vi "3-Position Solenoid Control.vi"(6 "Sensor Analog Status":sgl format="%#_13g", 7 "Sensor Digital Status":bool, 9 "Feedback":T5, 10 "Action":T4(ring), 11 "PneumaticsDevRefIn":T1={"Pneumatic State Reference"=refnum, "SolenoidDevRef"={"DevStatus"={"status"=FALSE, "code"=0, "source"=""}, "Pneumatics Control Module"=0, "Forward Solenoid Channel"=enum."Invalid", "Reverse Solenoid Channel"=enum."Invalid"}, "Pneumatic Configuration reference"=refnum}) -> (1 "Action Complete":bool, 2 "Forward":bool, 3 "PneumaticsDevRefOut":T1={"Pneumatic State Reference"=refnum, "SolenoidDevRef"={"DevStatus"={"status"=FALSE, "code"=0, "source"=""}, "Pneumatics Control Module"=0, "Forward Solenoid Channel"=enum."Invalid", "Reverse Solenoid Channel"=enum."Invalid"}, "Pneumatic Configuration reference"=refnum})   [LabVIEW 2015]
uses:
  <userlib>/836 Library/Pneumatics/Common/Feedback Typedef.ctl
  <userlib>/836 Library/Pneumatics/Pneumatics/836_PneumaticsDevRef.ctl
  <userlib>/836 Library/Pneumatics/Pneumatics/Pneumatic State.ctl
  <userlib>/836 Library/Pneumatics/Pneumatics/StateMachine.ctl
  <vilib>/Rock Robotics/WPI/Solenoid/WPI_SolenoidDevRef.ctl
  <vilib>/Rock Robotics/WPI/Solenoid/WPI_SolenoidChannel.ctl
  <userlib>/836 Library/Pneumatics/Pneumatics/Pneumatic Configuration.ctl
  <vilib>/Rock Robotics/WPI/Solenoid/WPI_SolenoidValue.ctl
  <vilib>/Rock Robotics/WPI/Solenoid/WPI_SolenoidSetEnum.vi
panel:
  out "error IO":errorcluster
  out "Error Out":errorcluster
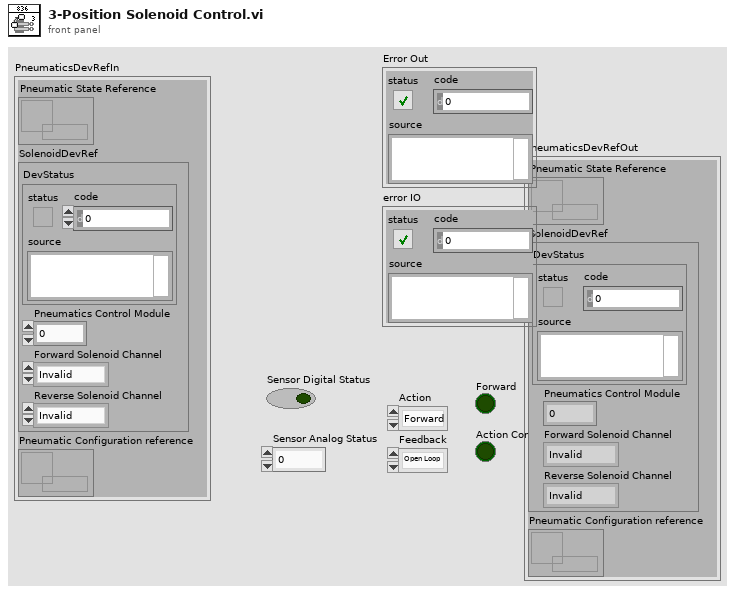
[diagram p1: front panel]
types:
  T1 = typedef "836_PneumaticsDevRef.ctl" = cluster{"Pneumatic State Reference":refnum<data-value>, "SolenoidDevRef":T2, "Pneumatic Configuration reference":refnum<data-value>}
  T2 = typedef "WPI_SolenoidDevRef.ctl" = cluster{"DevStatus":errorcluster, "Pneumatics Control Module":u8, "Forward Solenoid Channel":T3, "Reverse Solenoid Channel":T3}
  T3 = typedef "WPI_SolenoidChannel.ctl" = enum8{"Solenoid 0", "Solenoid 1", "Solenoid 2", "Solenoid 3", "Solenoid 4", "Solenoid 5", "Solenoid 6", "Solenoid 7", "Invalid"}
  T4 = enum16{"Forward", "Back", "Toggle", "Status", "Float"}
  T5 = typedef "Feedback Typedef.ctl" = enum16{"Open Loop", "Analog", "Digital", "Timed", "Digital Timeout"}
  T6 = typedef "WPI_SolenoidValue.ctl" = enum16{"Off", "On", "Forward", "Reverse"}
  T7 = typedef "StateMachine.ctl" = enum8{"Status", "Forward", "Back", "Toggle", "Timed Forward", "Timed Back", "Analog Forwad", "Analog Back", "Digital Forward", "Digital Back", "Off", "Float", "Digital Forward Timeout", "Digital Back Timeout"}
  T8 = typedef "Pneumatic State.ctl" = cluster{"Position":bool, "Initialize":bool, "Current State":T7, "Multiuse Timer A":u32, "Multiuse Timer B":u32}
  T9 = typedef "Pneumatic Configuration.ctl" = cluster{"Time Forward (ms)":u32, "Time Back (ms)":u32, "Digital Forward Time (ms)":u32, "Digital Backward Time (ms)":u32, "Analog Forward Settling Time (ms)":u32, "Analog Backward Settling Time (ms)":u32, "Analog Forward Threshold":sgl, "Analog Backward Threshold":sgl}
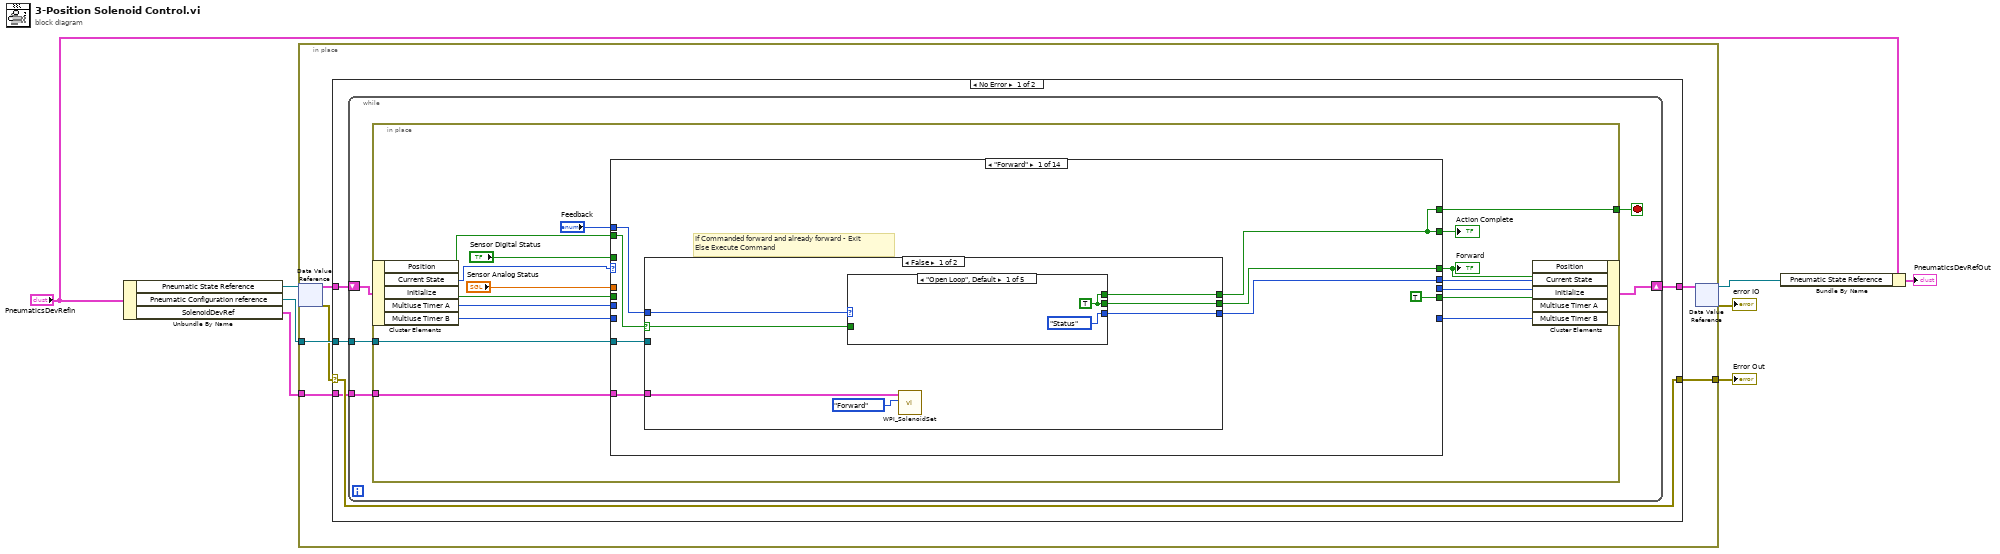
[diagram p0: block diagram]
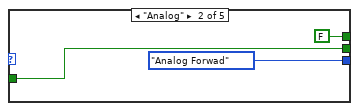
[diagram p2: hidden frame]
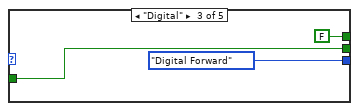
[diagram p3: hidden frame]
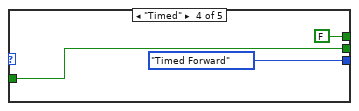
[diagram p4: hidden frame]
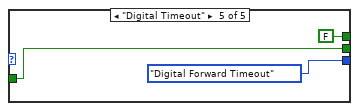
[diagram p5: hidden frame]
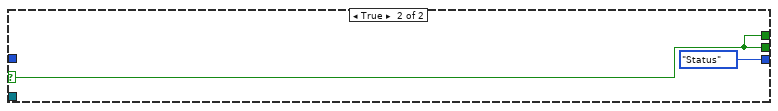
[diagram p6: hidden frame]
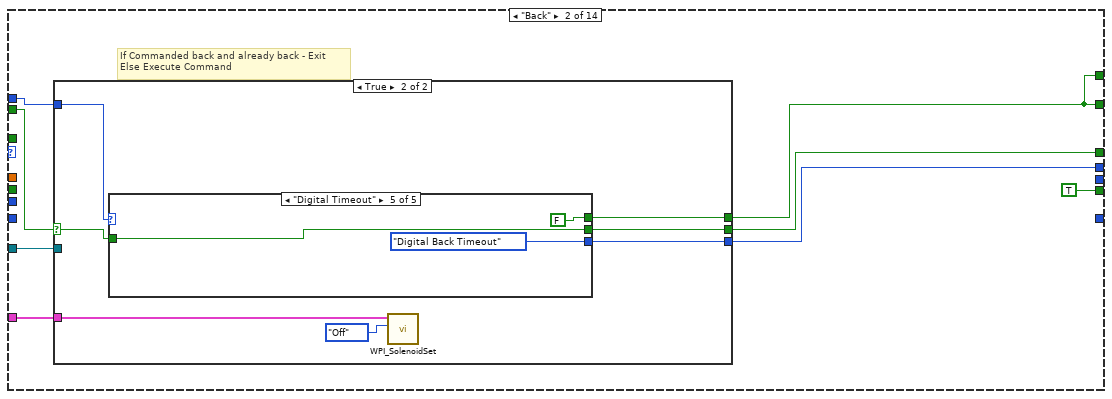
[diagram p7: hidden frame]
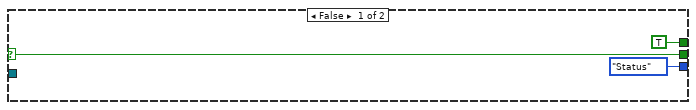
[diagram p8: hidden frame]
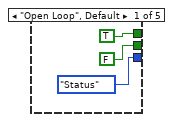
[diagram p9: hidden frame]
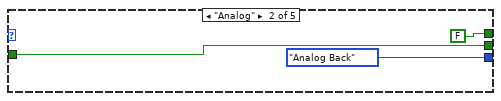
[diagram p10: hidden frame]
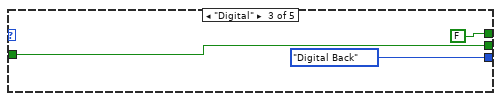
[diagram p11: hidden frame]
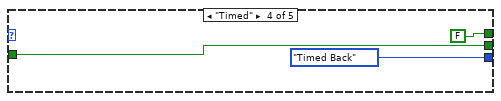
[diagram p12: hidden frame]
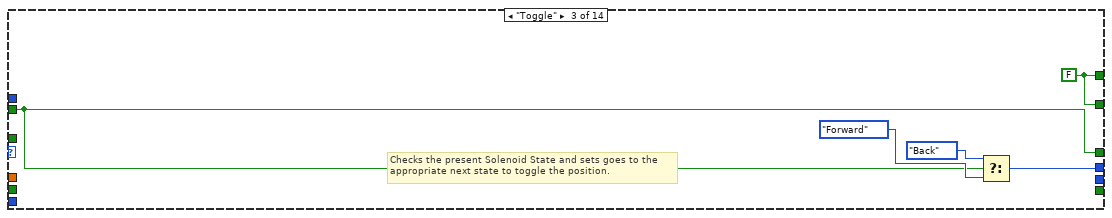
[diagram p13: hidden frame]
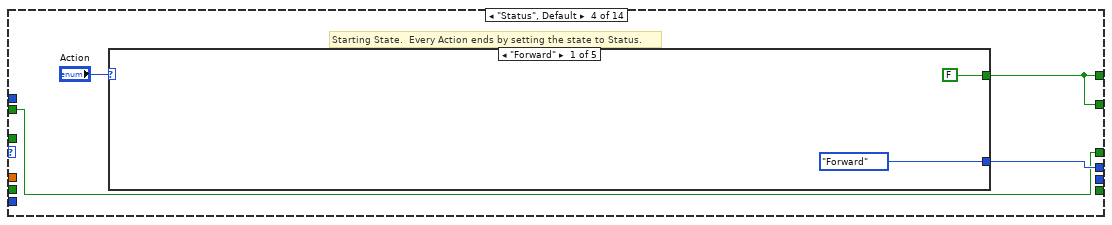
[diagram p14: hidden frame]
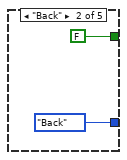
[diagram p15: hidden frame]
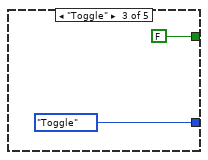
[diagram p16: hidden frame]
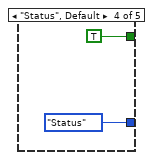
[diagram p17: hidden frame]
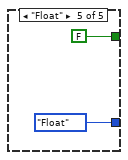
[diagram p18: hidden frame]
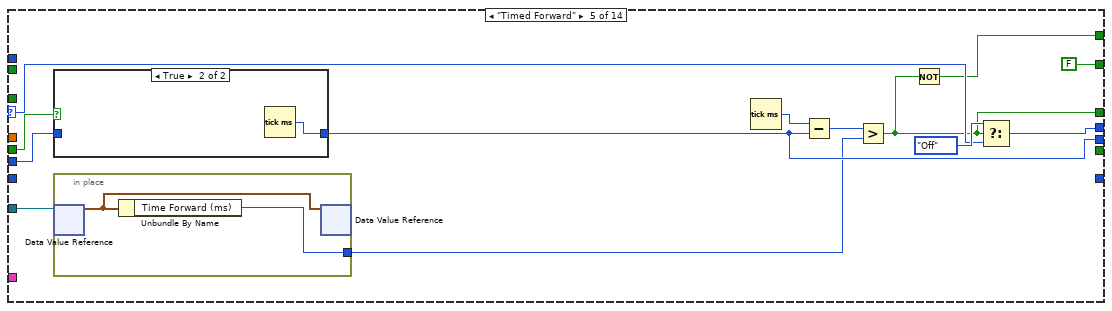
[diagram p19: hidden frame]
diagram:
  n1 = Unbundle By Name("PneumaticsDevRefIn") -> ("Pneumatic State Reference"=w8:refnum<data-value>, "Pneumatic Configuration reference"=w7:refnum<data-value>, "SolenoidDevRef"=w1:T2)
  n2 = in-place {
    in-place-border: w7 -> [w13]
    in-place-border: [w10] -> w3
    in-place-border: w1 -> [w9]
    n3 = in-place-dvr #1(w8) -> (w14:T8, w11:errorcluster)
    n4 = case shown="No Error" w11 {
      selector: w11 -> [w17 w292]
      tunnel: w14 -> [w19 w293]
      tunnel: w13 -> [w18 _]
      tunnel: [w16 w293] -> w12
      tunnel: [w17 w292] -> w10
      tunnel: w9 -> [w15 _]
      frame No Error {
        n5 = while {
          tunnel: w18 -> [w23]
          shift-right: [w21] -> w16
          shift-left: w19 -> [w24]
          tunnel: w15 -> [w20]
          stop <- w22 stop-if-true
          n6 = in-place {
            in-place-border: w23 -> [w33]
            in-place-border: [w29] -> w22
            in-place-border: w20 -> [w27]
            n7 = in-place-cluster #2(w24) -> ("Position"=w37:bool, "Current State"=w31:T7, "Initialize"=w36:bool, "Multiuse Timer A"=w32:u32, "Multiuse Timer B"=w26:u32)
            n8 = case shown="\"Forward\"" w31 {
              selector: w31 -> [_ _ _ _ w135 w150 w167 w192 w212 w235 w250 w271 _ _]
              tunnel: [w47 w78 w106 w112 w127 w144 w162 w183 w203 w228 w245 w264 w282 w289] -> w29
              tunnel: "Feedback" -> [w49 w80 _ _ _ _ _ _ _ _ _ _ _ _]
              tunnel: w37 -> [w45 w77 w109 w113 _ _ _ _ _ _ _ _ w283 w290]
              tunnel: [w48 w79 w109 w113 w128 w144 w161 w183 w204 w220 w245 w264 w283 w290] -> w35
              tunnel: "Sensor Digital Status" -> [_ _ _ _ _ _ _ _ w214 w237 w253 w274 _ _]
              tunnel: [w46 w76 w107 w114 w136 w153 w174 w195 w215 w238 w254 w275 StateMachine."Status" StateMachine."Status"] -> w34
              tunnel: "Sensor Analog Status" -> [_ _ _ _ _ _ w171 w189 _ _ _ _ _ _]
              tunnel: w36 -> [_ _ _ _ w129 w145 w163 w184 w206 w223 w246 w260 _ _]
              tunnel: [w47 w78 w106 w112 FALSE FALSE FALSE FALSE FALSE FALSE FALSE FALSE w282 w289] -> w38
              tunnel: w32 -> [_ _ _ _ w130 w146 w164 w185 w207 w230 w247 w268 _ _]
              tunnel: [_ _ _ _ w131 w147 w165 w186 w208 w231 w248 w269 _ _] -> w28
              tunnel: w33 -> [w44 w75 _ _ w126 w143 w160 w182 w202 w227 w244 w267 _ _]
              tunnel: [TRUE TRUE _ _ _ _ _ _ _ _ _ _ _ _] -> w30
              tunnel: w27 -> [w42 w73 _ _ _ _ _ _ _ _ _ _ w281 w288]
              tunnel: w26 -> [_ _ _ _ _ _ _ _ _ w225 _ w261 _ _]
              tunnel: [_ _ _ _ _ _ _ _ _ w222 _ w262 _ _] -> w25
              frame "Forward" {
                # "If Commanded forward and already forward - Exit\nElse Execute Command"
                n9 = case shown="False" w45 {
                  selector: w45 -> [w52 w71]
                  tunnel: w49 -> [w56 _]
                  tunnel: [w55 w71] -> w48
                  tunnel: [w54 w71] -> w47
                  tunnel: [w53 StateMachine."Status"] -> w46
                  tunnel: w44 -> [_ _]
                  tunnel: w42 -> [w50 _]
                  frame False {
                    n10 = case shown="\"Open Loop\", Default" w56 {
                      tunnel: [w57 FALSE FALSE FALSE FALSE] -> w54
                      tunnel: [StateMachine."Status" StateMachine."Analog Forwad" StateMachine."Digital Forward" StateMachine."Timed Forward" StateMachine."Digital Forward Timeout"] -> w53
                      tunnel: w52 -> [_ w59 w62 w65 w70]
                      tunnel: [w57 w59 w62 w65 w70] -> w55
                      frame "Open Loop", Default {
                        w57 = TRUE
                      }
                      frame "Analog" {
                      }
                      frame "Digital" {
                      }
                      frame "Timed" {
                      }
                      frame "Digital Timeout" {
                      }
                    }
                    n11 = call-poly <vilib>:"WPI_SolenoidSet.vi"("Value"=WPI_SolenoidValue."Forward" ("Value 3"), "SolenoidDevRef"=w50) -> ()  [unwired: 8 in, 2 out]
                  }
                  frame True {
                  }
                }
              }
              frame "Back" {
                # "If Commanded back and already back - Exit\nElse Execute Command"
                n12 = case shown="True" w77 {
                  selector: w77 -> [w81 w86]
                  tunnel: w80 -> [_ w90]
                  tunnel: [w81 w89] -> w79
                  tunnel: [TRUE w88] -> w78
                  tunnel: [StateMachine."Status" w87] -> w76
                  tunnel: w75 -> [_ _]
                  tunnel: w73 -> [_ w84]
                  frame False {
                  }
                  frame True {
                    n13 = case shown="\"Digital Timeout\"" w90 {
                      tunnel: [TRUE FALSE FALSE FALSE FALSE] -> w88
                      tunnel: [StateMachine."Status" StateMachine."Analog Back" StateMachine."Digital Back" StateMachine."Timed Back" StateMachine."Digital Back Timeout"] -> w87
                      tunnel: [FALSE w94 w97 w100 w103] -> w89
                      tunnel: w86 -> [_ w94 w97 w100 w103]
                      frame "Open Loop", Default {
                      }
                      frame "Analog" {
                      }
                      frame "Digital" {
                      }
                      frame "Timed" {
                      }
                      frame "Digital Timeout" {
                      }
                    }
                    n14 = call-poly <vilib>:"WPI_SolenoidSet.vi"("Value"=WPI_SolenoidValue."Off" ("Value 3"), "SolenoidDevRef"=w84) -> ()  [unwired: 8 in, 2 out]
                  }
                }
              }
              frame "Toggle" {
                w106 = FALSE
                # "Checks the present Solenoid State and sets goes to the\nappropriate next state to toggle the position."
                n15 = Select(t=StateMachine."Back", s=w109, f=StateMachine."Forward") -> (s? t:f=w107:T7)
              }
              frame "Status", Default {
                # "Starting State.  Every Action ends by setting the state to Status."
                n16 = case shown="\"Forward\"" "Action" {
                  tunnel: [FALSE FALSE FALSE TRUE FALSE] -> w112
                  tunnel: [StateMachine."Forward" StateMachine."Back" StateMachine."Toggle" StateMachine."Status" StateMachine."Float"] -> w114
                  frame "Forward" {
                  }
                  frame "Back" {
                  }
                  frame "Toggle" {
                  }
                  frame "Status", Default {
                  }
                  frame "Float" {
                  }
                }
              }
              frame "Timed Forward" {
                n17 = case shown="True" w129 {
                  tunnel: [w140 w141] -> w131
                  tunnel: w130 -> [w140 _]
                  frame False {
                  }
                  frame True {
                    n18 = Tick Count (ms)() -> (millisecond timer value=w141:u32)
                  }
                }
                n19 = in-place {
                  in-place-border: [w138] -> w125
                  n20 = in-place-dvr #3(w126) -> (w139:T9)  [unwired: 1 out]
                  n21 = Unbundle By Name(w139) -> ("Time Forward (ms)"=w138:u32)
                  n22 = in-place-dvr #3(w139) -> ()  [unwired: 2 out]
                }
                n23 = Tick Count (ms)() -> (millisecond timer value=w133:u32)
                n24 = Subtract(x=w133, y=w131) -> (x-y=w134:u32)
                n25 = Greater?(x=w134, y=w125) -> (0:w128:bool)
                n26 = Not(x=w128) -> (.not. x?=w127:bool)
                n27 = Select(t=StateMachine."Off", s=w128, f=w135) -> (s? t:f=w136:T7)
              }
              frame "Timed Back" {
                n28 = case shown="True" w145 {
                  tunnel: [w156 w157] -> w147
                  tunnel: w146 -> [w156 _]
                  frame False {
                  }
                  frame True {
                    n29 = Tick Count (ms)() -> (millisecond timer value=w157:u32)
                  }
                }
                n30 = in-place {
                  in-place-border: [w154] -> w142
                  n31 = in-place-dvr #4(w143) -> (w155:T9)  [unwired: 1 out]
                  n32 = Unbundle By Name(w155) -> ("Time Back (ms)"=w154:u32)
                  n33 = in-place-dvr #4(w155) -> ()  [unwired: 2 out]
                }
                n34 = Tick Count (ms)() -> (millisecond timer value=w149:u32)
                n35 = Subtract(x=w149, y=w147) -> (x-y=w152:u32)
                n36 = Less Or Equal?(x=w152, y=w142) -> (x <= y?=w144:bool)
                n37 = Select(t=w150, s=w144, f=StateMachine."Off") -> (s? t:f=w153:T7)
              }
              frame "Analog Forwad" {
                n38 = in-place {
                  in-place-border: [w176] -> w159
                  in-place-border: [w175] -> w158
                  n39 = in-place-dvr #5(w160) -> (w177:T9)  [unwired: 1 out]
                  n40 = Unbundle By Name(w177) -> ("Analog Forward Settling Time (ms)"=w176:u32, "Analog Forward Threshold"=w175:sgl)
                  n41 = in-place-dvr #5(w177) -> ()  [unwired: 2 out]
                }
                n42 = Greater?(x=w158, y=w171) -> (0:w170:bool)
                n43 = Or(x=w170, y=w163) -> (x .or. y?=w172:bool)
                n44 = case shown="True" w172 {
                  tunnel: [w178 w179] -> w165
                  tunnel: w164 -> [w178 _]
                  frame False {
                  }
                  frame True {
                    n45 = Tick Count (ms)() -> (millisecond timer value=w179:u32)
                  }
                }
                n46 = Tick Count (ms)() -> (millisecond timer value=w173:u32)
                n47 = Subtract(x=w173, y=w165) -> (x-y=w169:u32)
                n48 = Greater?(x=w169, y=w159) -> (0:w161:bool)
                n49 = Not(x=w161) -> (.not. x?=w162:bool)
                n50 = Select(t=StateMachine."Off", s=w161, f=w167) -> (s? t:f=w174:T7)
              }
              frame "Analog Back" {
                n51 = in-place {
                  in-place-border: [w197] -> w181
                  in-place-border: [w196] -> w180
                  n52 = in-place-dvr #6(w182) -> (w198:T9)  [unwired: 1 out]
                  n53 = Unbundle By Name(w198) -> ("Analog Backward Threshold"=w197:sgl, "Analog Backward Settling Time (ms)"=w196:u32)
                  n54 = in-place-dvr #6(w198) -> ()  [unwired: 2 out]
                }
                n55 = Greater Or Equal?(x=w189, y=w181) -> (x >= y?=w188:bool)
                n56 = Or(x=w184, y=w188) -> (x .or. y?=w190:bool)
                n57 = case shown="True" w190 {
                  tunnel: [w199 w200] -> w186
                  tunnel: w185 -> [w199 _]
                  frame False {
                  }
                  frame True {
                    n58 = Tick Count (ms)() -> (millisecond timer value=w200:u32)
                  }
                }
                n59 = Tick Count (ms)() -> (millisecond timer value=w191:u32)
                n60 = Subtract(x=w191, y=w186) -> (x-y=w194:u32)
                n61 = Less?(x=w194, y=w180) -> (x < y?=w183:bool)
                n62 = Select(t=w192, s=w183, f=StateMachine."Off") -> (s? t:f=w195:T7)
              }
              frame "Digital Forward" {
                n63 = in-place {
                  in-place-border: [w217] -> w201
                  n64 = in-place-dvr #7(w202) -> (w218:T9)  [unwired: 1 out]
                  n65 = Unbundle By Name(w218) -> ("Digital Forward Time (ms)"=w217:u32)
                  n66 = in-place-dvr #7(w218) -> ()  [unwired: 2 out]
                }
                n67 = Not(x=w206) -> (.not. x?=w205:bool)
                n68 = And(x=w214, y=w205) -> (x .and. y?=w213:bool)
                n69 = Increment(x=w207) -> (x+1=w210:u32)
                n70 = Select(t=w210, s=w213, f=u32 0 ("t")) -> (s? t:f=w208:u32)
                n71 = Greater Or Equal?(x=w208, y=w201) -> (x >= y?=w204:bool)
                n72 = Not(x=w204) -> (.not. x?=w203:bool)
                n73 = Select(t=StateMachine."Off", s=w204, f=w212) -> (s? t:f=w215:T7)
              }
              frame "Digital Forward Timeout" {
                n74 = in-place {
                  in-place-border: [w241] -> w226
                  in-place-border: [w240] -> w224
                  n75 = in-place-dvr #8(w227) -> (w242:T9)  [unwired: 1 out]
                  n76 = Unbundle By Name(w242) -> ("Digital Forward Time (ms)"=w241:u32, "Time Forward (ms)"=w240:u32)
                  n77 = in-place-dvr #8(w242) -> ()  [unwired: 2 out]
                }
                n78 = Not(x=w223) -> (.not. x?=w229:bool)
                n79 = And(x=w237, y=w229) -> (x .and. y?=w236:bool)
                n80 = Increment(x=w230) -> (x+1=w233:u32)
                n81 = Select(t=w233, s=w236, f=u32 0 ("t")) -> (s? t:f=w231:u32)
                n82 = Greater Or Equal?(x=w231, y=w226) -> (x >= y?=w220:bool)
                n83 = Not(x=w220) -> (.not. x?=w228:bool)
                n84 = call <userlib>:"Timer Embedded.vi"("Time Limit"=w224, "Reset"=w223, "Start Time In"=w225) -> ("Time Limit Passed"=w221:bool, "Start Time Out"=w222:u32)  [unwired: 7 in]
                n85 = Or(x=w220, y=w221) -> (x .or. y?=w219:bool)
                n86 = Select(t=StateMachine."Off", s=w219, f=w235) -> (s? t:f=w238:T7)
              }
              frame "Digital Back" {
                n87 = in-place {
                  in-place-border: [w257] -> w243
                  n88 = in-place-dvr #9(w244) -> (w258:T9)  [unwired: 1 out]
                  n89 = Unbundle By Name(w258) -> ("Digital Backward Time (ms)"=w257:u32)
                  n90 = in-place-dvr #9(w258) -> ()  [unwired: 2 out]
                }
                n91 = Not Or(1:w253, 2:w246) -> (0:w255:bool)
                n92 = Increment(x=w247) -> (x+1=w252:u32)
                n93 = Select(t=w252, s=w255, f=u32 0 ("t")) -> (s? t:f=w248:u32)
                n94 = Less?(x=w248, y=w243) -> (x < y?=w245:bool)
                n95 = Select(t=w250, s=w245, f=StateMachine."Off") -> (s? t:f=w254:T7)
              }
              frame "Digital Back Timeout" {
                n96 = in-place {
                  in-place-border: [w279] -> w266
                  in-place-border: [w278] -> w259
                  n97 = in-place-dvr #10(w267) -> (w280:T9)  [unwired: 1 out]
                  n98 = Unbundle By Name(w280) -> ("Digital Backward Time (ms)"=w279:u32, "Time Back (ms)"=w278:u32)
                  n99 = in-place-dvr #10(w280) -> ()  [unwired: 2 out]
                }
                n100 = Not Or(1:w274, 2:w260) -> (0:w276:bool)
                n101 = Increment(x=w268) -> (x+1=w273:u32)
                n102 = Select(t=w273, s=w276, f=u32 0 ("t")) -> (s? t:f=w269:u32)
                n103 = Less?(x=w269, y=w266) -> (x < y?=w264:bool)
                n104 = call <userlib>:"Timer Embedded.vi"("Time Limit"=w259, "Reset"=w260, "Start Time In"=w261) -> ("Time Limit Passed"=w265:bool, "Start Time Out"=w262:u32)  [unwired: 7 in]
                n105 = Or(x=w264, y=w265) -> (x .or. y?=w263:bool)
                n106 = Select(t=w271, s=w263, f=StateMachine."Off") -> (s? t:f=w275:T7)
              }
              frame "Off" {
                w282 = TRUE
                # "Disabled so this VI can be used for 3-Position Solenoids"
                n107 = disable-structure shown="Disabled" {
                  disable-tunnel: w281 -> [w285 _]
                  frame Disabled {
                    n108 = call-poly <vilib>:"WPI_SolenoidSet.vi"("Value"=WPI_SolenoidValue."Off" ("Value 3"), "SolenoidDevRef"=w285) -> ()  [unwired: 8 in, 2 out]
                  }
                  frame Enabled {
                  }
                }
              }
              frame "Float" {
                w289 = TRUE
                n109 = call-poly <vilib>:"WPI_SolenoidSet.vi"("Value"=WPI_SolenoidValue."Off" ("Value 3"), "SolenoidDevRef"=w288) -> ()  [unwired: 8 in, 2 out]
              }
            }
            "Forward" <- w35
            "Action Complete" <- w38
            n110 = in-place-cluster #2("Position"=w35, "Current State"=w34, "Initialize"=w30, "Multiuse Timer A"=w28, "Multiuse Timer B"=w25) -> (w21:T8)
          }
        }
      }
      frame Error {
      }
    }
    n111 = in-place-dvr #1(w12) -> (w4:refnum<data-value>, →"error IO":errorcluster)
  }
  "Error Out" <- w3
  n112 = Bundle By Name(cluster="PneumaticsDevRefIn", "Pneumatic State Reference"=w4) -> (→"PneumaticsDevRefOut":T1)
